vi "Send Start Vision.vi"(7 "Message Priority (Normal)":T2=enum."Normal", 8 "error in (no error)":errorcluster, 10 "Input":T1, 11 "Message Enqueuer":refnum<class "Message Enqueuer.lvclass">) -> (0 "error out":errorcluster, 3 "Message Enqueuer out":refnum<class "Message Enqueuer.lvclass">)   [LabVIEW 2022 SP3, in "Start Vision Msg 2.lvclass"]
doc: "This VI sends the message to an actor."
uses:
  Start Vision Msg 2.lvclass
  <vilib>/ActorFramework/Message Enqueuer/Message Enqueuer.lvclass
  <vilib>/ActorFramework/Message Enqueuer/Message Priority.ctl
  UDP Input.ctl
  C:/Program Files (x86)/National Instruments/LabVIEW 2022/vi.lib/ActorFramework/Message/Message.lvclass
  Start Vision Msg 2.lvclass/Start Vision Msg 2.ctl
  <vilib>/ActorFramework/Message Enqueuer/Message Enqueuer.lvclass/Message Enqueuer.ctl
  <vilib>/ActorFramework/Message Priority Queue/Priority Enqueue.vi
  C:/Users/ebert/Documents/codes/ssl/repo/Phoenix Reborn/UDP Data Receiver/UDP Data Receiver Messages/Start Vision Msg/Start Vision Msg 2.lvclass
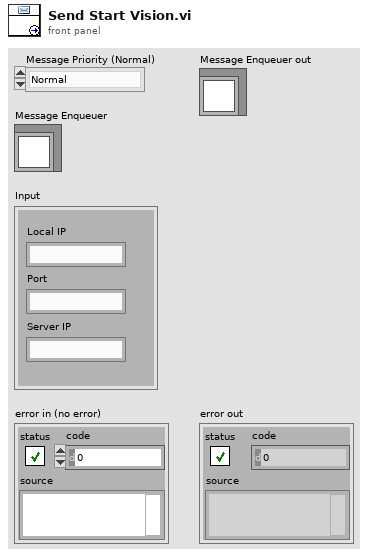
[diagram p1: front panel]
types:
  T1 = typedef "UDP Input.ctl" = cluster{"Local IP":string, "Port":string, "Server IP":string}
  T2 = typedef "Actor Framework.lvlib/Message Enqueuer.lvclass/Message Priority.ctl" = enum16{"Low", "Normal", "High"}
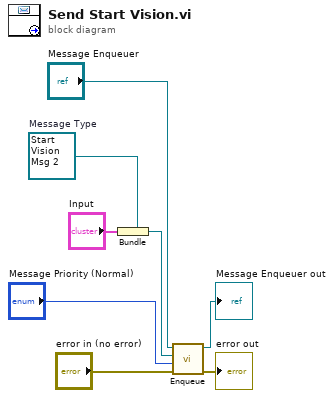
[diagram p0: block diagram]
diagram:
  w5 = refnum<class "Start Vision Msg 2.lvclass"> refnum  # Message Type
  n1 = Bundle(cluster=w5, "Input") -> (w4:refnum<class "Start Vision Msg 2.lvclass">)
  n2 = call <vilib>:"Enqueue.vi"("error in (no error)"="error in (no error)", "Message Priority (Normal)"="Message Priority (Normal)", "Message"=w4, "Message Enqueuer in"="Message Enqueuer") -> ("error out"=→"error out":errorcluster, "Message Enqueuer in"=→"Message Enqueuer out":refnum<class "Message Enqueuer.lvclass">)  [unwired: 6 in]
